vi "Time-out wait loop helper.vi"(9 "Time-out (ms)":u32, 10 "Done?":bool, 11 "Time-out value in":u32) -> (1 "Timed out?":bool, 2 "Done or timed out?":bool, 3 "Time-out value out":u32)   [LabVIEW 2014, in "COSYLib.lvlib"]
doc: "Helper VI for waiting loops that feature a time-out.\nDrop this VI inside a while loop, and wire the \"Time-out value\" terminals to a U32 shift register that's initialized to 0. Wire the \"Done or timed out?\" output terminal to the \"Stop\" terminal of the while loop. This helper VI will now take care of the time-out logic."
uses:
  COSYLib.lvlib
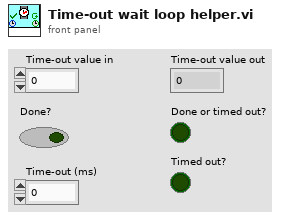
[diagram p1: front panel]
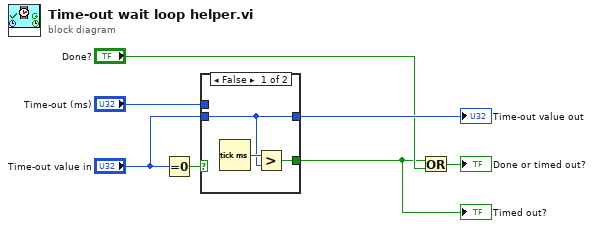
[diagram p0: block diagram]
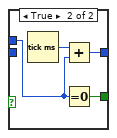
[diagram p2: hidden frame]
diagram:
  n1 = Equal To 0?(x="Time-out value in") -> (x = 0?=w7:bool)
  n2 = case shown="False" w7 {
    tunnel: "Time-out (ms)" -> [_ w11]
    tunnel: [w9 w13] -> w5
    tunnel: "Time-out value in" -> [w9 _]
    tunnel: [w8 w12] -> w2
    frame False {
      n3 = Tick Count (ms)() -> (millisecond timer value=w10:u32)
      n4 = Greater?(x=w10, y=w9) -> (0:w8:bool)
    }
    frame True {
      n5 = Tick Count (ms)() -> (millisecond timer value=w14:u32)
      n6 = Add(x=w14, y=w11) -> (x+y=w13:u32)
      n7 = Equal To 0?(x=w11) -> (x = 0?=w12:bool)
    }
  }
  "Timed out?" <- w2
  "Time-out value out" <- w5
  n8 = Or(x=w2, y="Done?") -> (x .or. y?=→"Done or timed out?":bool)
